vi "Begin.vi"() -> (0 "error out":errorcluster)   [LabVIEW 2013]
doc: "Called before other user functions, this VI is expected to open initial I/O refnums, load in file data, and do all program initialization. Notice that the <B>error out</B> terminal is simply used for data flow. Wiring it to other structures or subVIs ensures that this VI runs first."
uses:
  <vilib>/Rock Robotics/SystemInterfaces/DIO/FPGA_DIOPWMChannel.ctl
  <vilib>/Rock Robotics/WPI/DriverStation/WPI_DriverStationRobotMode2.ctl
  <vilib>/Rock Robotics/WPI/Joystick/WPI_JoystickDeviceEnum.ctl
  <vilib>/Rock Robotics/SystemInterfaces/AI/FPGA_AIChannel.ctl
  <vilib>/Rock Robotics/WPI/SafetyOutput/WPI_SafetyOutputConfigMenu.ctl
  <vilib>/Rock Robotics/SystemInterfaces/DIO/FPGA_DIORelayChannel.ctl
  <vilib>/Rock Robotics/WPI/Solenoid/WPI_SolenoidChannel.ctl
  <vilib>/Rock Robotics/SystemInterfaces/DIO/FPGA_DIOChannel.ctl
  <vilib>/Rock Robotics/WPI/Relay/WPI_RelayDirection.ctl
  <vilib>/Rock Robotics/WPI/Encoder/WPI_EncoderType.ctl
  <vilib>/Rock Robotics/WPI/RobotDrive/WPI_RobotDriveOpen2MotorWithVictor.vi
  Robot Global Data.vi
  <vilib>/Rock Robotics/WPI/MotorControl/WPI_MotorControlOpen Talon.vi
  <vilib>/Rock Robotics/WPI/Counter/WPI_CounterDigitalInputToDigitalSource.vi
  <vilib>/Rock Robotics/WPI/Solenoid/WPI_SolenoidOpenDouble.vi
panel:
  out "error out 2":errorcluster
  out "EncoderError":errorcluster[](array[cluster])
  out "WOTMotor":errorcluster
  out "WOTErrors":errorcluster[](array[cluster])
  out "Shooter Relay Errors":errorcluster[](array[cluster])
  out "error out 3":errorcluster
  out "Back Ultrasonic Error?":errorcluster
  out "Front Ultrasonic Error?":errorcluster
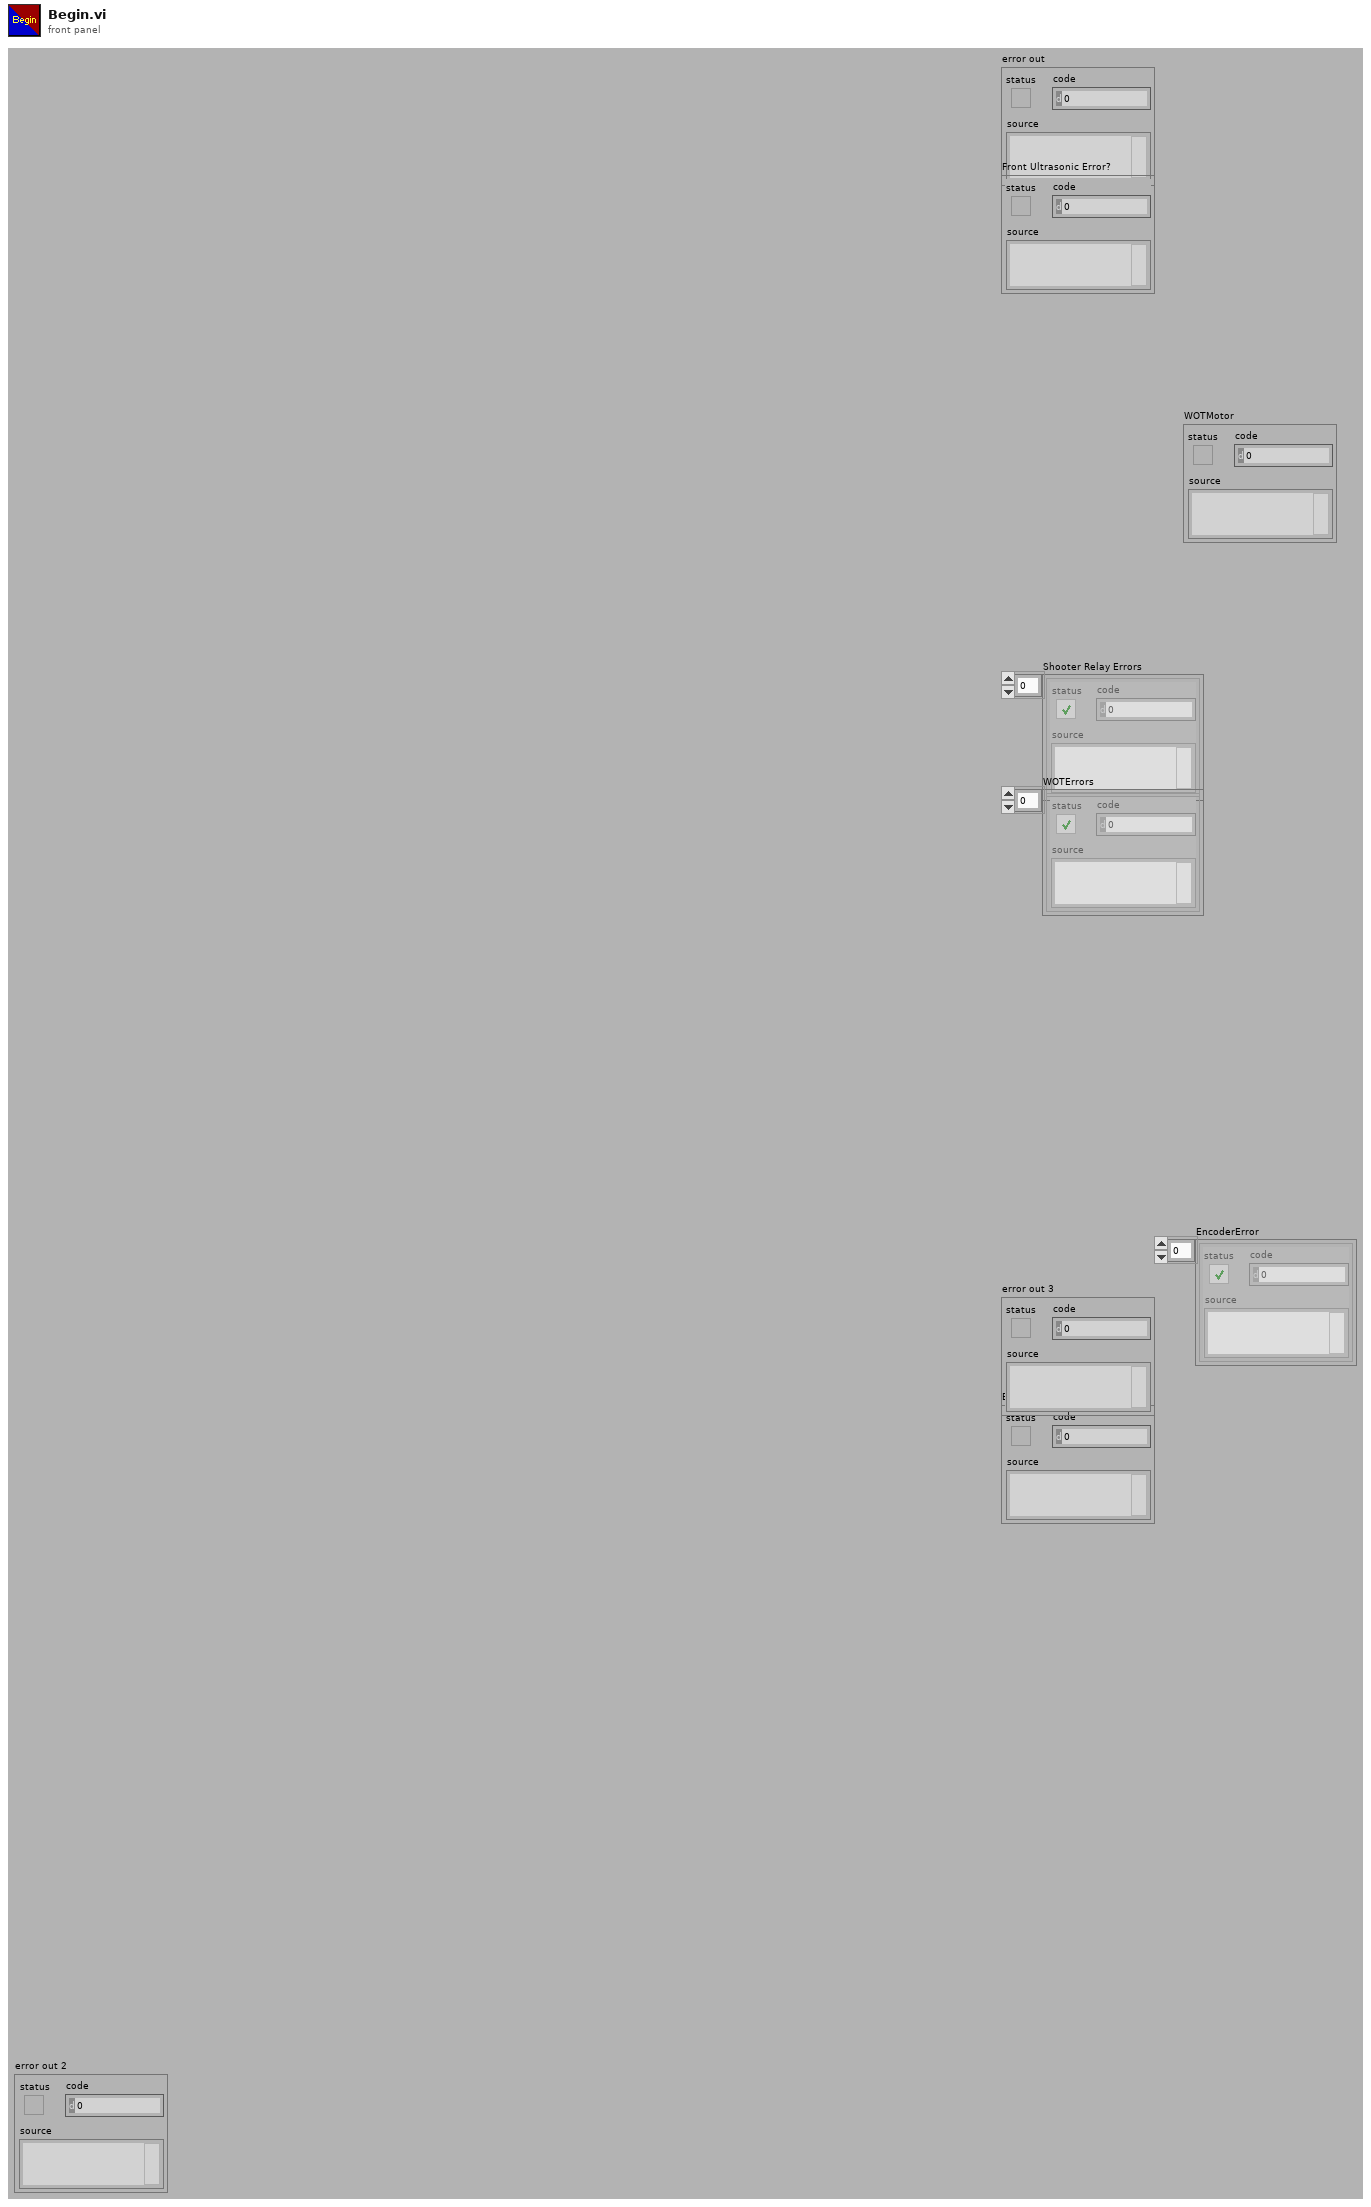
[diagram p1: front panel]
types:
  T1 = typedef "WPI_JoystickDeviceEnum.ctl" = enum16{"USB 1", "USB 2", "USB 3", "USB 4", "Kinect 1", "Kinect 2"}
  T2 = typedef "FPGA_DIOChannel.ctl" = enum8{"DIO 1", "DIO 2", "DIO 3", "DIO 4", "DIO 5", "DIO 6", "DIO 7", "DIO 8", "DIO 9", "DIO 10", "DIO 11", "DIO 12", "DIO 13", "DIO 14", "Invalid"}
  T3 = cluster{"refnum name":string, "DIO Channel":T2, "DIO Channel 2":T2}[]
  T4 = typedef "WPI_SolenoidChannel.ctl" = enum8{"Solenoid 1", "Solenoid 2", "Solenoid 3", "Solenoid 4", "Solenoid 5", "Solenoid 6", "Solenoid 7", "Solenoid 8", "Invalid"}
  T5 = cluster{string, "Solenoid Channel":T4, "Solenoid Channel 2":T4}[]
  T6 = typedef "FPGA_DIORelayChannel.ctl" = enum8{"Relay 1", "Relay 2", "Relay 3", "Relay 4", "Relay 5", "Relay 6", "Relay 7", "Relay 8", "Invalid"}
  T7 = cluster{"refnum name":string, "Relay Channel":T6}[]
  T8 = typedef "WPI_SafetyOutputConfigMenu.ctl" = enum16{"Enable", "Disable"}
  T9 = typedef "FPGA_DIOPWMChannel.ctl" = enum8{"PWM 1", "PWM 2", "PWM 3", "PWM 4", "PWM 5", "PWM 6", "PWM 7", "PWM 8", "PWM 9", "PWM 10", "Invalid"}
  T10 = typedef "FPGA_AIChannel.ctl" = enum8{"AI 1", "AI 2", "AI 3", "AI 4", "AI 5", "AI 6", "AI 7", "AI 8", "Invalid"}
  T11 = typedef "WPI_DriverStationRobotMode2.ctl" = enum16{"Autonomous Disabled", "Autonomous Enabled", "Teleop Disabled", "Teleop Enabled", "Timeout", "Finish", "Test Disabled", "Test Enabled"}
  T12 = typedef "WPI_JoystickDevRef.ctl" = cluster{"Device":T1}
  T13 = typedef "WPI_AnalogChannelDevRef.ctl" = cluster{"DevStatus":errorcluster, "Analog Module":T14, "Analog Channel":T10}
  T14 = typedef "FPGA_TypedefAnalogModule.ctl" = enum16{"Analog Module 1", "Analog Module 2"}
  T15 = typedef "WPI_MotorControlDeviceRef.ctl" = cluster{"DeviceStatus":errorcluster, "Type":enum16{"PWM", "CAN"}, "PWM":cluster{"Digital Module":T16, "PWM Channel":T9, "DeadBand":T17}, "CAN":cluster{"Device Number":u8, "Control Mode":T18, "Semaphore":T19, "Max Vout":dbl}, "Invert":bool, "TransformRef":T20, "InvTransformRef":T20}
  T16 = typedef "FPGA_TypedefDigitalModule.ctl" = enum16{"Digital Module 1", "Digital Module 2"}
  T17 = typedef "WPI_PWMDeadband.ctl" = cluster{"Name":string, "maxPositivePwm":i32, "minPositivePwm":i32, "centerPwm":i32, "maxNegativePwm":i32, "minNegativePwm":i32, "angularRange":u16}
  T18 = typedef "WPI_CANJaguar_ControlMode.ctl" = enum8{"Percent VBus", "Current", "Speed", "Position", "Voltage"}
  T19 = typedef "Semaphore RefNum" = refnum<k1>
  T20 = typedef "WPI_PWMTransform_ConPane.ctl" = refnum<vi>
  T21 = typedef "WPI_RelayDirection.ctl" = enum16{"Both directions", "Forward only", "Reverse only"}
  T22 = typedef "WPI_RelayDevRef.ctl" = cluster{"DevStatus":errorcluster, "Relay Channel":T6, "Digital Module":T16, "Relay Direction":T21}
  T23 = typedef "WPI_EncoderType.ctl" = enum16{"1x", "2x", "4x"}
  T24 = typedef "WPI_DigitalInputDevRef.ctl" = cluster{"DevStatus":errorcluster, "DIO Channel":T2, "Digital Module":T16}
  T25 = typedef "FPGA_CounterEncoderSourceConvertionLVSourceType.ctl" = cluster{"DevStatus":errorcluster, "AnalogTriggerMode?":bool, "DigitalMode":cluster{"Digital Module":T16, "DIO Channel":T26}, "AnalogTriggerMode":cluster{"AnalogTriggerIndex":T27, "OutputType":T28}}
  T26 = typedef "FPGA_DIODigitalSourceChannel.ctl" = enum8{"DIO 1", "DIO 2", "DIO 3", "DIO 4", "DIO 5", "DIO 6", "DIO 7", "DIO 8", "DIO 9", "DIO 10", "DIO 11", "DIO 12", "DIO 13", "DIO 14", "Disabled"}
  T27 = typedef "FPGA_AnalogTriggerIndex.ctl" = enum8{"Trig 0", "Trig 1", "Trig 2", "Trig 3", "Trig 4", "Trig 5", "Trig 6", "Trig 7", "Invalid"}
  T28 = typedef "FPGA_AnalogTriggerOutType.ctl" = enum16{"InWindow", "TriggerState", "Rising", "Falling"}
  T29 = typedef "WPI_EncoderDevRef.ctl" = cluster{"DevStatus":errorcluster, "EncoderIndex":T30, "CounterIndex":T31, "DistancePerCount":dbl, "Decoding Type":T23}
  T30 = typedef "FPGA_EncoderIdx.ctl" = enum8{"Enc 0", "Enc 1", "Enc 2", "Enc 3", "Invalid"}
  T31 = typedef "FPGA_CounterCtrSystemIndex.ctl" = enum8{"Ctr 0", "Ctr 1", "Ctr 2", "Ctr 3", "Ctr 4", "Ctr 5", "Ctr 6", "Ctr 7", "Invalid"}
  T32 = typedef "WPI_SolenoidDevRef.ctl" = cluster{"DevStatus":errorcluster, "Solenoid Module":T33, "Forward Solenoid Channel":T4, "Reverse Solenoid Channel":T4}
  T33 = typedef "FPGA_TypedefSolenoidModule.ctl" = enum16{"Solenoid Module 1", "Solenoid Module 2"}
  T34 = typedef "WPI_RobotDriveDevRef.ctl" = cluster{"DevStatus":errorcluster, "Motors[]":T15[], "Square Inputs":bool, "Max Output":dbl, "Isochronous":bool}
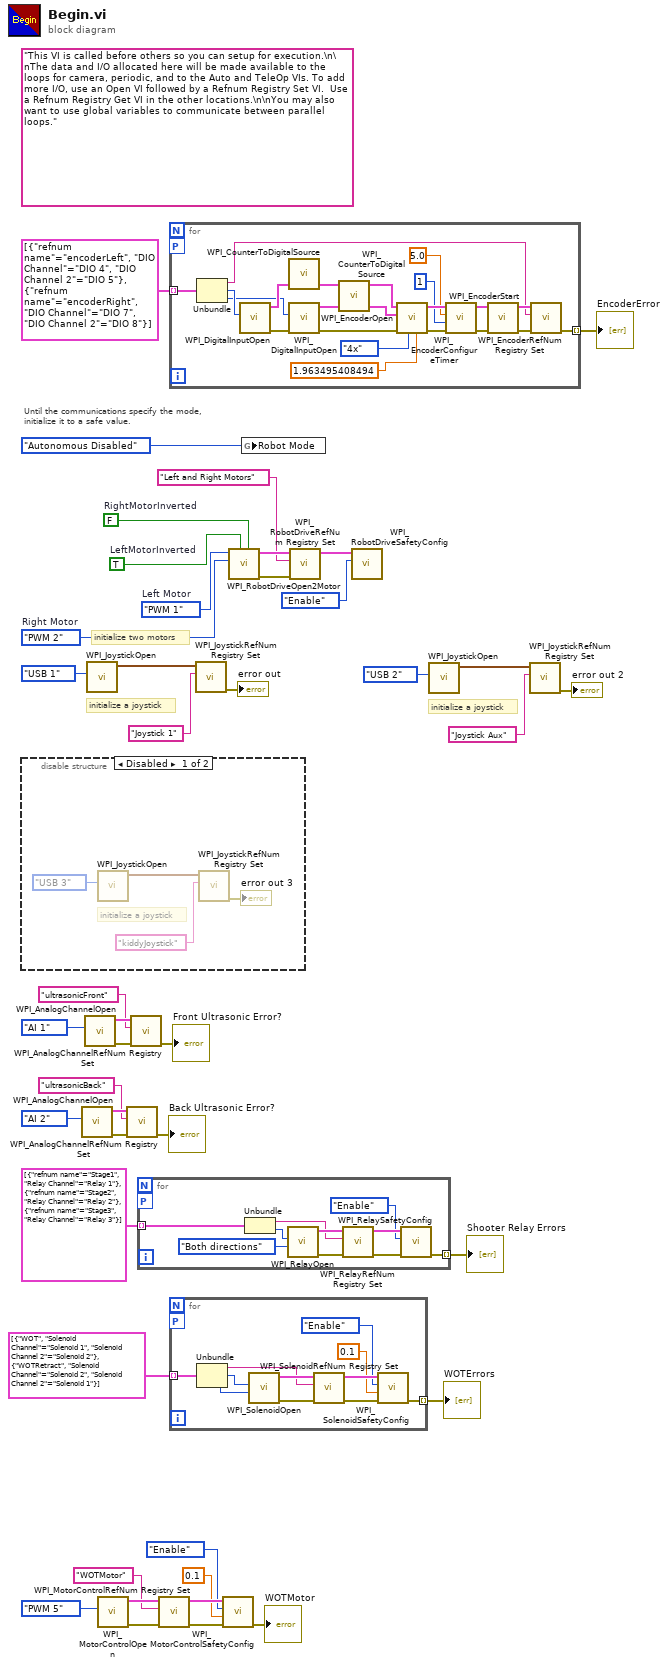
[diagram p0: block diagram]
diagram:
  (unwired) "This VI is called before others so you can setup for execution.\n\nThe data and I/O allocated here will be made available to the loops for camera, periodic, and to the Auto and TeleOp VIs. To add more I/O, use an Open VI followed by a Refnum Registry Set VI.  Use a Refnum Registry Get VI in the other locations.\n\nYou may also want to use global variables to communicate between parallel loops."
  w37 = FPGA_DIOPWMChannel."PWM 2"  # Right Motor
  w38 = FPGA_DIOPWMChannel."PWM 1"  # Left Motor
  w42 = TRUE  # LeftMotorInverted
  w43 = FALSE  # RightMotorInverted
  # "initialize a joystick"
  # "initialize a joystick"
  # "Until the communications specify the mode,\ninitialize it to a safe value."
  # "initialize two motors"
  n1 = disable-structure shown="Disabled" {
    frame Disabled {
      # "initialize a joystick"
      n2 = call <vilib>:"WPI_JoystickOpen.vi"("JoystickDevice"=WPI_JoystickDeviceEnum."USB 3") -> ("JoystickDevRef"=w46:T12)  [unwired: 10 in]
      n3 = call <vilib>:"WPI_JoystickRefNum Registry Set.vi"("refnum name"="kiddyJoystick", "JoystickDevRef"=w46) -> ("error out"=→"error out 3":errorcluster)  [unwired: 8 in, 1 out]
    }
    frame Enabled {
    }
  }
  n4 = call <vilib>:"WPI_AnalogChannelOpen.vi"("Analog Channel"=FPGA_AIChannel."AI 2") -> ("error out"=w22:errorcluster, "AIDeviceRef"=w23:T13)  [unwired: 9 in]
  n5 = call <vilib>:"WPI_AnalogChannelOpen.vi"("Analog Channel"=FPGA_AIChannel."AI 1") -> ("error out"=w27:errorcluster, "AIDeviceRef"=w28:T13)  [unwired: 9 in]
  n6 = call <vilib>:"WPI_JoystickOpen.vi"("JoystickDevice"=WPI_JoystickDeviceEnum."USB 1") -> ("JoystickDevRef"=w32:T12)  [unwired: 10 in]
  n7 = call-poly <vilib>:"WPI_MotorControlOpen.vi"("PWM Channel"=FPGA_DIOPWMChannel."PWM 5") -> ("error out"=w11:errorcluster, "MotorControlDeviceRef"=w16:T15)  [unwired: 9 in]
  n8 = call <vilib>:"WPI_AnalogChannelRefNum Registry Set.vi"("error in (no error)"=w22, "refnum name"="ultrasonicBack", "AIDeviceRef"=w23) -> ("error out"=→"Back Ultrasonic Error?":errorcluster)  [unwired: 7 in, 1 out]
  n9 = call <vilib>:"WPI_AnalogChannelRefNum Registry Set.vi"("error in (no error)"=w27, "refnum name"="ultrasonicFront", "AIDeviceRef"=w28) -> ("error out"=→"Front Ultrasonic Error?":errorcluster)  [unwired: 7 in, 1 out]
  n10 = for {
    tunnel: [w51] -> w19 mode=indexing
    tunnel: T7 [{"refnum name"="Stage1", "Relay Channel"=enum."Relay 1"}, {"refnum name"="Stage2", "Relay Channel"=enum."Relay 2"}, {"refnum name"="Stage3", "Relay Channel"=enum."Relay 3"}] -> [w50] mode=indexing
    workers-P: _ -> [_]
    n11 = Unbundle(w50) -> ("refnum name"=w49:string, "Relay Channel"=w48:T6)
    n12 = call <vilib>:"WPI_RelayOpen.vi"("Relay Direction"=WPI_RelayDirection."Both directions", "Relay Channel"=w48) -> ("error out"=w55:errorcluster, "RelayDevRef"=w56:T22)  [unwired: 8 in]
    n13 = call <vilib>:"WPI_RelayRefNum Registry Set.vi"("error in (no error)"=w55, "refnum name"=w49, "RelayDevRef"=w56) -> ("error out"=w53:errorcluster, "RelayDevRef"=w54:T22)  [unwired: 7 in]
    n14 = call <vilib>:"WPI_RelaySafetyConfig.vi"("error in (no error)"=w53, "mode"=WPI_SafetyOutputConfigMenu."Enable", "RelayDevRef"=w54) -> ("error out"=w51:errorcluster)  [unwired: 7 in, 1 out]
  }
  "Shooter Relay Errors" <- w19
  n15 = call <vilib>:"WPI_MotorControlRefNum Registry Set.vi"("error in (no error)"=w11, "refnum name"="WOTMotor", "MotorControlDevRef"=w16) -> ("error out"=w10:errorcluster, "MotorControlDevRef"=w14:T15)  [unwired: 7 in]
  n16 = for {
    tunnel: [w62] -> w5 mode=indexing
    tunnel: T3 [{"refnum name"="encoderLeft", "DIO Channel"=enum."DIO 4", "DIO Channel 2"=enum."DIO 5"}, {"refnum name"="encoderRight", "DIO Channel"=enum."DIO 7", "DIO Channel 2"=enum."DIO 8"}] -> [w58] mode=indexing
    workers-P: _ -> [_]
    n17 = Unbundle(w58) -> ("refnum name"=w59:string, "DIO Channel"=w61:T2, "DIO Channel 2"=w60:T2)
    n18 = call <vilib>:"WPI_DigitalInputOpen.vi"("DIO Channel"=w61) -> ("error out"=w78:errorcluster, "DigitalInputDevRef"=w77:T24)  [unwired: 9 in]
    n19 = call-poly <vilib>:"WPI_CounterToDigitalSource.vi"("DigitalInputDevRef"=w77) -> ("Digital Source"=w75:T25)  [unwired: 6 in]
    n20 = call <vilib>:"WPI_DigitalInputOpen.vi"("error in (no error)"=w78, "DIO Channel"=w60) -> ("error out"=w71:errorcluster, "DigitalInputDevRef"=w76:T24)  [unwired: 8 in]
    n21 = call-poly <vilib>:"WPI_CounterToDigitalSource.vi"("DigitalInputDevRef"=w76) -> ("Digital Source"=w74:T25)  [unwired: 6 in]
    n22 = call <vilib>:"WPI_EncoderOpen.vi"("DistancePerCount"=1.963495408494, "Decoding Type"=WPI_EncoderType."4x", "error in (no error)"=w71, "BSource"=w74, "ASource"=w75) -> ("error out"=w69:errorcluster, "EncoderDevRef"=w70:T29)  [unwired: 5 in]
    n23 = call <vilib>:"WPI_EncoderConfigureTimer.vi"("error in (no error)"=w69, "Number Samples to Average"=u8 1, "Minimum Rate"=5.0, "EncoderDevRef"=w70) -> ("error out"=w65:errorcluster, "EncoderDevRef"=w66:T29)  [unwired: 6 in]
    n24 = call <vilib>:"WPI_EncoderStart.vi"("error in (no error)"=w65, "EncoderDevRef"=w66) -> ("error out"=w63:errorcluster, "EncoderDevRef"=w64:T29)  [unwired: 8 in]
    n25 = call <vilib>:"WPI_EncoderRefNum Registry Set.vi"("error in (no error)"=w63, "refnum name"=w59, "EncoderDevRef"=w64) -> ("error out"=w62:errorcluster)  [unwired: 7 in, 1 out]
  }
  "EncoderError" <- w5
  n26 = for {
    tunnel: [w83] -> w18 mode=indexing
    tunnel: T5 [{"WOT", "Solenoid Channel"=enum."Solenoid 1", "Solenoid Channel 2"=enum."Solenoid 2"}, {"WOTRetract", "Solenoid Channel"=enum."Solenoid 2", "Solenoid Channel 2"=enum."Solenoid 1"}] -> [w82] mode=indexing
    workers-P: _ -> [_]
    n27 = Unbundle(w82) -> (w81:string, "Solenoid Channel"=w80:T4, "Solenoid Channel 2"=w79:T4)
    n28 = call-poly <vilib>:"WPI_SolenoidOpen.vi"("Reverse Solenoid Channel"=w79, "Forward Solenoid Channel"=w80) -> ("error out"=w85:errorcluster, "SolenoidDevRef"=w89:T32)  [unwired: 2 in, 6 out]
    n29 = call <vilib>:"WPI_SolenoidRefNum Registry Set.vi"("error in (no error)"=w85, "refnum name"=w81, "SolenoidDevRef"=w89) -> ("error out"=w84:errorcluster, "SolenoidDevRef"=w88:T32)  [unwired: 7 in]
    n30 = call <vilib>:"WPI_SolenoidSafetyConfig.vi"("error in (no error)"=w84, "timeout (s)"=0.1, "mode"=WPI_SafetyOutputConfigMenu."Enable", "SolenoidDevRef"=w88) -> ("error out"=w83:errorcluster)  [unwired: 6 in, 1 out]
  }
  "WOTErrors" <- w18
  n31 = call <vilib>:"WPI_JoystickRefNum Registry Set.vi"("refnum name"="Joystick 1", "JoystickDevRef"=w32) -> ("error out"=→"error out":errorcluster)  [unwired: 8 in, 1 out]
  n32 = call <vilib>:"WPI_MotorControlSafetyConfig.vi"("error in (no error)"=w10, "timeout (s)"=0.1, "mode"=WPI_SafetyOutputConfigMenu."Enable", "MotorControlDevRef"=w14) -> ("error out"=→"WOTMotor":errorcluster)  [unwired: 6 in, 1 out]
  n33 = call-poly <vilib>:"WPI_RobotDriveOpen2Motor.vi"("Right Motor Inverted"=w43, "Left Motor Inverted"=w42, "Right Motor"=w37, "Left Motor"=w38) -> ("error out"=w39:errorcluster, "RobotDriveDevRef"=w41:T34)  [unwired: 1 in, 5 out]
  n34 = global write "Robot Global Data.vi" "Robot Mode"(WPI_DriverStationRobotMode2."Autonomous Disabled" ("Robot Mode")) -> ()
  n35 = call <vilib>:"WPI_RobotDriveRefNum Registry Set.vi"("error in (no error)"=w39, "refnum name"="Left and Right Motors", "RobotDriveDevRef"=w41) -> ("RobotDriveDevRef"=w36:T34)  [unwired: 8 out]
  n36 = call <vilib>:"WPI_RobotDriveSafetyConfig.vi"("mode"=WPI_SafetyOutputConfigMenu."Enable", "RobotDriveDevRef"=w36) -> ()  [unwired: 8 in, 2 out]
  n37 = call <vilib>:"WPI_JoystickOpen.vi"("JoystickDevice"=WPI_JoystickDeviceEnum."USB 2") -> ("JoystickDevRef"=w3:T12)  [unwired: 10 in]
  n38 = call <vilib>:"WPI_JoystickRefNum Registry Set.vi"("refnum name"="Joystick Aux", "JoystickDevRef"=w3) -> ("error out"=→"error out 2":errorcluster)  [unwired: 8 in, 1 out]
